vi "Differential.vi"(1 "Ts":dbl, 2 "X[k-1]":dbl, 3 "X[k]":dbl) -> (0 "dX":dbl)   [LabVIEW 2017]
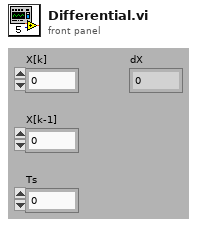
[diagram p1: front panel]
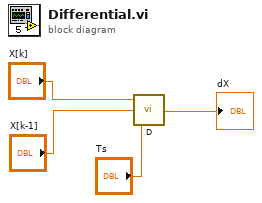
[diagram p0: block diagram]
diagram:
  n1 = call "D.vi"("Ts"="Ts", "e[k-1]"="X[k-1]", "e[k]"="X[k]") -> ("d"=→"dX":dbl)
